vi "Subtract - RM,RM.vi"(1 "Real Matrix B":T1, 2 "Real Matrix A":T1) -> (0 "A - B":T1)   [LabVIEW 2017, in "NI_Matrix.lvlib"]
doc: "Computes the difference of the inputs."
uses:
  NI_Matrix.lvlib
  RealMatrix.ctl
  Array To Matrix - RA2.vi
  Matrix To Array - RM.vi
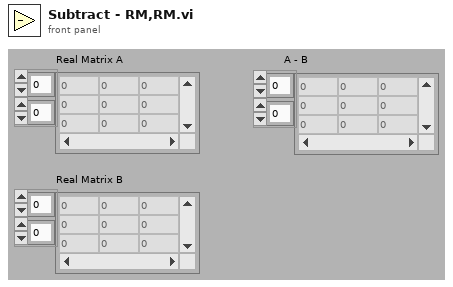
[diagram p1: front panel]
types:
  T1 = typedef "NI_Matrix.lvlib/RealMatrix.ctl" = dbl[][]
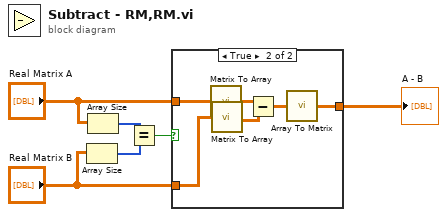
[diagram p0: block diagram]
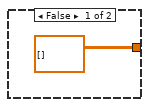
[diagram p2: hidden frame]
diagram:
  n1 = Array Size(array="Real Matrix B") -> (size(s)=w5:i32[])
  n2 = Array Size(array="Real Matrix A") -> (size(s)=w6:i32[])
  n3 = Equal?(x=w6, y=w5) -> (x = y?=w4:bool)
  n4 = case shown="True" w4 {
    tunnel: "Real Matrix A" -> [_ w12]
    tunnel: "Real Matrix B" -> [_ w13]
    tunnel: [T1 [] ("A - B") w8] -> w1
    frame False {
    }
    frame True {
      n5 = call-poly "Matrix To Array.vi"("Real Matrix"=w12) -> ("Real 2D Array"=w11:dbl[][])
      n6 = call-poly "Matrix To Array.vi"("Real Matrix"=w13) -> ("Real 2D Array"=w10:dbl[][])
      n7 = Subtract(x=w11, y=w10) -> (x-y=w9:dbl[][])
      n8 = call-poly "Array To Matrix.vi"("Real 2D Array"=w9) -> ("Real Matrix"=w8:T1)
    }
  }
  "A - B" <- w1
